vi "Measurement Logic.vi"() -> ()   [LabVIEW 2021, in "audio_acMeasurement.lvlib"]
uses:
  audio_acMeasurement.lvlib
  <vilib>/MeasurementLink/MeasurementLink Measurement Server/Classes/MeasurementContext/MeasurementContext.lvclass
  Measurement Results.ctl
  Measurement Configuration.ctl
  <vilib>/PDM Acquisition Toolkit/host/Classes/Tasks/PCM Input/Controls/DVR PCM Input Task.ctl
  <vilib>/PDM Acquisition Toolkit/host/Classes/Tasks/PCM Input/PCM Input Task.lvclass
  shared/controls/Protocol settings.ctl
  <vilib>/DAQmx/create/channels.llb/DAQmx Create Channel (AO-Voltage-Basic).vi
  <vilib>/DAQmx/configure/timing.llb/DAQmx Timing (Sample Clock).vi
  <vilib>/DAQmx/create/channels.llb/DAQmx Create Channel (AO-FuncGen).vi
  <vilib>/PDM Acquisition Toolkit/host/API/Public/Start/Start PCM Input Task.vi
  <vilib>/PDM Acquisition Toolkit/host/API/Public/Read/Read PCM Input Waveform.vi
  <vilib>/PDM Acquisition Toolkit/host/API/Public/Clear/Clear PCM Input Task.vi
  <resource>/objmgr/daqmx.rc
  <vilib>/PDM Acquisition Toolkit/host/API/PDM Acquisition Toolkit.lvlib
panel:
  in  "Measurement Configuration":T1={"Band start"=20.0, "Band stop"=20000.0, "Weighting filter"=0, "Full scale range"=3.16, "Analog source resource name"="", "Frequency"=1000.0, "Amplitude"=1.0, "Protocol capture resource name"="", "Protocol"="", "Clock rate"=12288000, "Number of words"=19200, "Sensitivity"=0.34762} {"Number of words" format="%#_6f"}
  out "Measurement Results":T2
  out "Measurement Context out":refnum<class "MeasurementContext.lvclass">
  in  "Measurement Context":refnum<class "MeasurementContext.lvclass">
  out "error out":errorcluster
  in  "error in":errorcluster
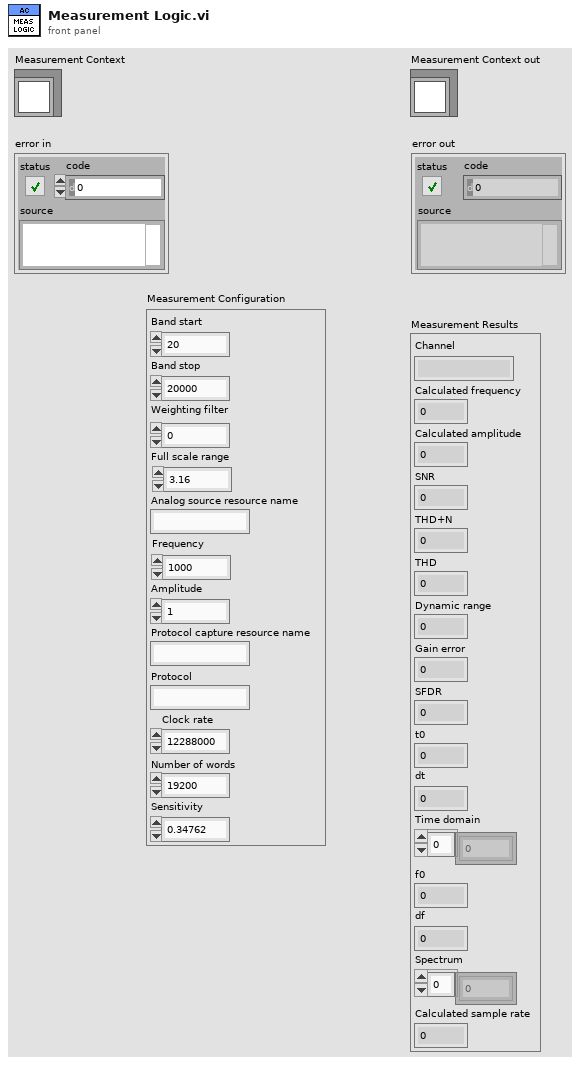
[diagram p1: front panel]
types:
  T1 = typedef "audio_acMeasurement.lvlib/Measurement Configuration.ctl" = cluster{"Band start":dbl, "Band stop":dbl, "Weighting filter":u16, "Full scale range":dbl, "Analog source resource name":string, "Frequency":dbl, "Amplitude":dbl, "Protocol capture resource name":string, "Protocol":string, "Clock rate":u32, "Number of words":i32, "Sensitivity":dbl}
  T2 = typedef "audio_acMeasurement.lvlib/Measurement Results.ctl" = cluster{"Channel":string, "Calculated frequency":dbl, "Calculated amplitude":dbl, "SNR":dbl, "THD+N":dbl, "THD":dbl, "Dynamic range":dbl, "Gain error":dbl, "SFDR":dbl, "t0":dbl, "dt":dbl, "Time domain":dbl[], "f0":dbl, "df":dbl, "Spectrum":dbl[], "Calculated sample rate":u32}
  T3 = typedef "PDM Acquisition Class Library.lvlib/PCM Input Task.lvclass/DVR PCM Input Task.ctl" = refnum<data-value>
  T4 = cluster{"DSG Session":refnum<k21>, "PDM task":T3}
  T5 = typedef "Protocol settings.ctl" = cluster{"Protocol capture resource name":string, "Clock rate":u32, "Number of words":i32, "Sensitivity":dbl, "Protocol":string}
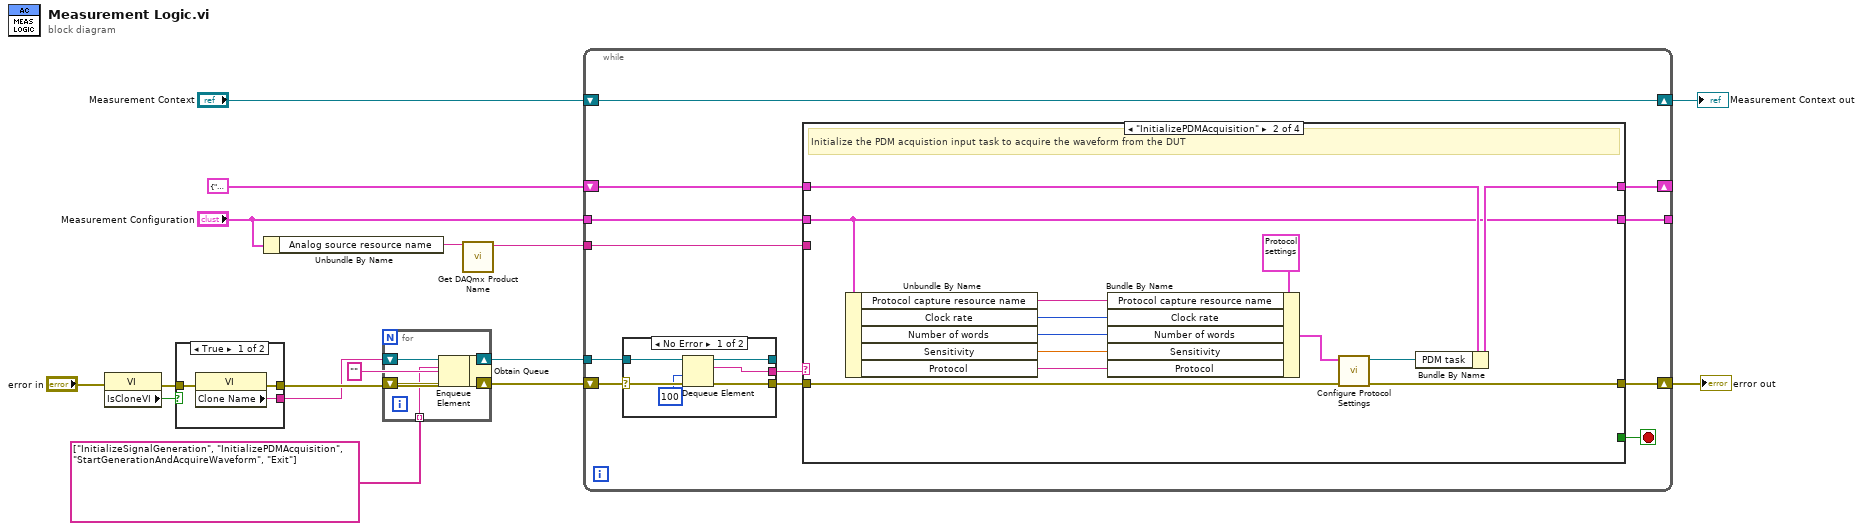
[diagram p0: block diagram]
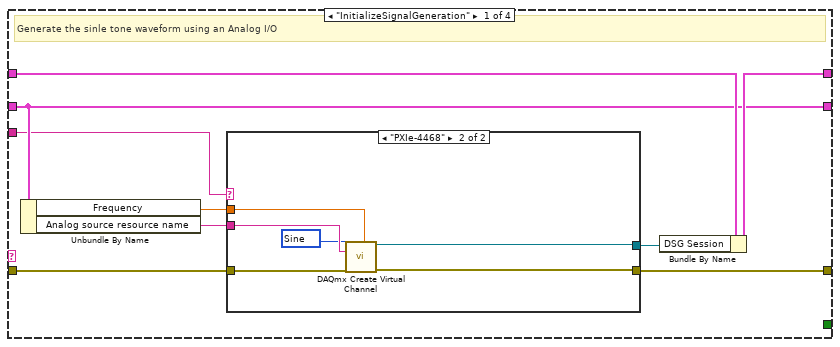
[diagram p2: hidden frame]
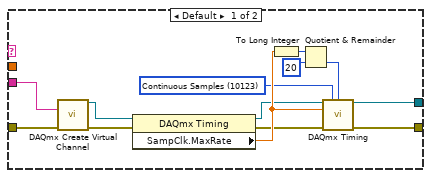
[diagram p3: hidden frame]
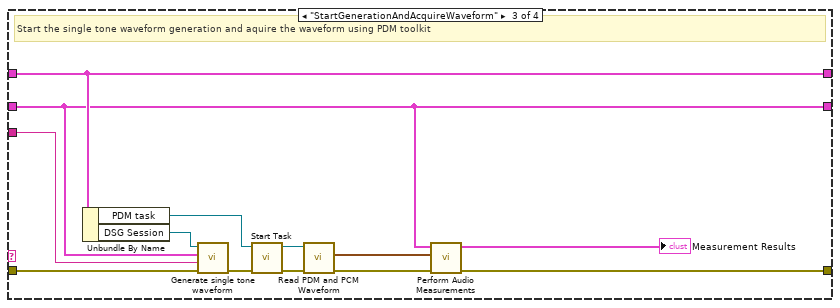
[diagram p4: hidden frame]
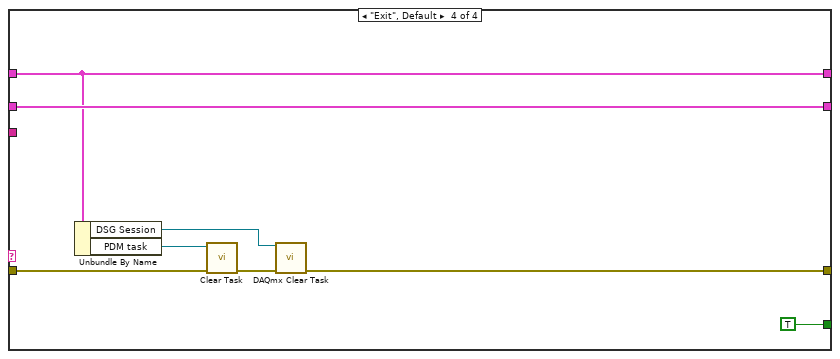
[diagram p5: hidden frame]
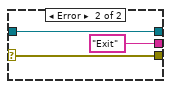
[diagram p6: hidden frame]
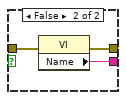
[diagram p7: hidden frame]
diagram:
  n1 = property class="VI"(error in="error in") -> (error out=w15:errorcluster, "IsCloneVI"=w16:bool)  [unwired: 1 in, 1 out]
  n2 = case shown="True" w16 {
    tunnel: [w21 w24] -> w14
    tunnel: [w20 w23] -> w13
    tunnel: w15 -> [w19 w22]
    frame True {
      n3 = property class="VI"(error in=w19) -> (error out=w21:errorcluster, "Clone Name"=w20:string)  [unwired: 1 in, 1 out]
    }
    frame False {
      n4 = property class="VI"(error in=w22) -> (error out=w24:errorcluster, "Name"=w23:string)  [unwired: 1 in, 1 out]
    }
  }
  n5 = Unbundle By Name("Measurement Configuration") -> ("Analog source resource name"=w5:string)
  n6 = Obtain Queue(name (unnamed)=w13, element data type="", error in (no error)=w14) -> (queue out=w17:refnum<queue>, error out=w12:errorcluster)  [unwired: 2 in, 1 out]
  n7 = for {
    shift-right: [w27] -> w11
    shift-left: w17 -> [w29]
    shift-right: [w26] -> w10
    shift-left: w12 -> [w28]
    tunnel: string[] ["InitializeSignalGeneration", "InitializePDMAcquisition", "StartGenerationAndAcquireWaveform", "Exit"] ("Step sequence") -> [w25] mode=indexing
    n8 = Enqueue Element(queue=w29, element=w25, error in (no error)=w28) -> (queue out=w27:refnum<queue>, error out=w26:errorcluster)  [unwired: 1 in, 1 out]
  }
  n9 = call "Get DAQmx Product Name.vi"("DAQmx resource name"=w5) -> ("DAQmx product type"=w4:string)  [unwired: 10 in]
  n10 = while {
    tunnel: w11 -> [w41]
    shift-right: [w38] -> w2
    shift-left: w10 -> [w37]
    shift-right: [w33] -> w6
    shift-left: "Measurement Context" -> [w33]
    tunnel: "Measurement Configuration" -> [w34]
    tunnel: [w35] -> _
    shift-right: [w31] -> _
    shift-left: T4 {"DSG Session"="", "PDM task"=refnum} -> [w36]
    tunnel: w4 -> [w30]
    stop <- w32 stop-if-true
    n11 = case shown="No Error" w37 {
      selector: w37 -> [w107 w111]
      tunnel: w41 -> [w109 w110]
      tunnel: [w108 "Exit" ("t")] -> w40
      tunnel: [w106 w111] -> w39
      tunnel: [w104 w110] -> _
      frame No Error {
        n12 = Dequeue Element(queue=w109, timeout in ms (-1)=100, error in (no error)=w107) -> (queue out=w104:refnum<queue>, element=w108:string, error out=w106:errorcluster)  [unwired: 1 out]
      }
      frame Error {
      }
    }
    n13 = case shown="\"InitializePDMAcquisition\"" w40 {
      tunnel: w39 -> [w49 w72 w91 w102]
      tunnel: [w48 w80 w88 w100] -> w38
      tunnel: w34 -> [w45 w78 w83 w103]
      tunnel: w36 -> [w47 w82 w86 w99]
      tunnel: [w46 w81 w86 w99] -> w31
      tunnel: [w45 w78 w83 w103] -> w35
      tunnel: [_ _ _ TRUE] -> w32
      tunnel: w30 -> [w43 _ w84 _]
      frame "InitializeSignalGeneration" {
        # "Generate the sinle tone waveform using an Analog I/O"
        n14 = Unbundle By Name(w45) -> ("Frequency"=w44:dbl, "Analog source resource name"=w50:string)
        n15 = case shown="\"PXIe-4468\"" w43 {
          tunnel: w50 -> [w63 w67]
          tunnel: w49 -> [w62 w69]
          tunnel: [w61 w68] -> w48
          tunnel: [w51 w64] -> w42
          tunnel: w44 -> [_ w65]
          frame Default {
            w52 = 10123 items=["Finite Samples"=10178, "Continuous Samples"=10123, "Hardware Timed Single Point"=12522] ("sample mode")
            n16 = call-poly <vilib>:"DAQmx Create Virtual Channel.vi"("physical channels"=w63, "error in"=w62) -> ("task out"=w60:refnum<k21>, "error out"=w59:errorcluster)  [unwired: 12 in]
            n17 = property class="DAQmx Timing"(reference=w60, error in=w59) -> (reference out=w55:refnum<k21>, error out=w56:errorcluster, "SampClk.MaxRate"=w57:dbl)
            n18 = To Long Integer(number=w57) -> (32bit integer=w53:i32)
            n19 = Quotient & Remainder(x=w53, y=20) -> (floor(x/y)=w58:i32)  [unwired: 1 out]
            n20 = call-poly <vilib>:"DAQmx Timing.vi"("task/channels in"=w55, "sample mode"=w52, "samples per channel"=w58, "rate"=w57, "error in"=w56) -> ("task out"=w51:refnum<k21>, "error out"=w61:errorcluster)  [unwired: 9 in]
          }
          frame "PXIe-4468" {
            w66 = 14751 items=["Sine"=14751, "Triangle"=14752, "Square"=14753, "Sawtooth"=14754] ("type")
            n21 = call-poly <vilib>:"DAQmx Create Virtual Channel.vi"("frequency"=w65, "physical channels"=w67, "type"=w66, "error in"=w69) -> ("task out"=w64:refnum<k21>, "error out"=w68:errorcluster)  [unwired: 10 in]
          }
        }
        n22 = Bundle By Name(cluster=w47, "DSG Session"=w42) -> (w46:T4)
      }
      frame "InitializePDMAcquisition" {
        # "Initialize the PDM acquistion input task to acquire the waveform from the DUT"
        n23 = Unbundle By Name(w78) -> ("Protocol capture resource name"=w71:string, "Clock rate"=w76:u32, "Number of words"=w75:i32, "Sensitivity"=w74:dbl, "Protocol"=w73:string)
        n24 = Bundle By Name(cluster=T5 {"Protocol capture resource name"="", "Clock rate"=12288000, "Number of words"=19200, "Sensitivity"=0.34762, "Protocol"=""} ("Protocol settings"), "Protocol capture resource name"=w71, "Clock rate"=w76, "Number of words"=w75, "Sensitivity"=w74, "Protocol"=w73) -> (w77:T5)
        n25 = call "Configure Protocol Settings.vi"("error in"=w72, "Protocol settings"=w77) -> ("error out"=w80:errorcluster, "PDM task"=w79:T3)  [unwired: 8 in]
        n26 = Bundle By Name(cluster=w82, "PDM task"=w79) -> (w81:T4)
      }
      frame "StartGenerationAndAcquireWaveform" {
        # "Start the single tone waveform generation and aquire the waveform using PDM toolkit"
        n27 = Unbundle By Name(w86) -> ("PDM task"=w92:T3, "DSG Session"=w90:refnum<k21>)
        n28 = call "Generate single tone waveform.vi"("error in"=w91, "DAQmx product type"=w84, "Measurement Configuration"=w83, "DSG task in"=w90) -> ("error out"=w93:errorcluster)  [unwired: 6 in, 1 out]
        n29 = call-poly <vilib>:"Start Task.vi"("error in"=w93, "PCM input task in"=w92) -> ("error out"=w95:errorcluster, "PCM input task out"=w94:T3)  [unwired: 8 in]
        n30 = call-poly <vilib>:"Read PDM and PCM Waveform.vi"("error in"=w95, "PCM input task In"=w94) -> ("error out"=w89:errorcluster, "PCM waveforms"=w87:waveform(dbl)[])  [unwired: 6 in, 2 out]
        n31 = call "Perform Audio Measurements.vi"("Measurement Configuration"=w83, "I2S waveforms"=w87, "error in"=w89) -> ("Measurement Results"=→"Measurement Results":T2, "error out"=w88:errorcluster)  [unwired: 6 in]
      }
      frame "Exit", Default {
        n32 = Unbundle By Name(w99) -> ("DSG Session"=w98:refnum<k21>, "PDM task"=w97:T3)
        n33 = call-poly <vilib>:"Clear Task.vi"("error in"=w102, "PCM input task in"=w97) -> ("error out"=w101:errorcluster)  [unwired: 9 in]
        n34 = call <vilib>:"DAQmx Clear Task.vi"("task in"=w98, "error in"=w101) -> ("error out"=w100:errorcluster)  [unwired: 13 in]
      }
    }
  }
  "error out" <- w2
  "Measurement Context out" <- w6
